vi "backwash.vi"(4 "Manual override":bool, 6 "Backwash control":T1, 8 "min filtration time [s]":dbl=600.0, 9 "Ripen time [s]":dbl=600.0, 10 "Filtered quality target [NTU]":dbl=0.3, 11 "Filtered Turbidity":dbl) -> (0 "backwashing?":i16, 1 "backwashing?":bool, 3 "last backwash":timestamp)   [LabVIEW 2019]
uses:
  Manual or Auto.ctl
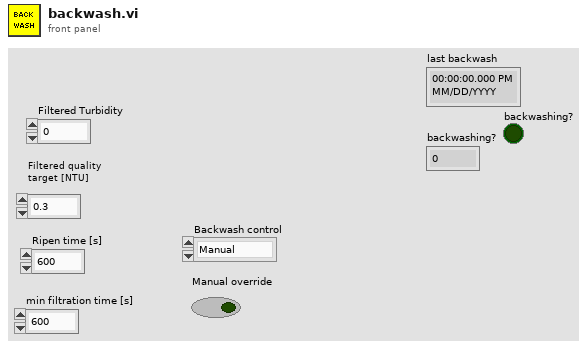
[diagram p1: front panel]
types:
  T1 = typedef "Manual or Auto.ctl" = enum16{"Manual", "Automatic"}
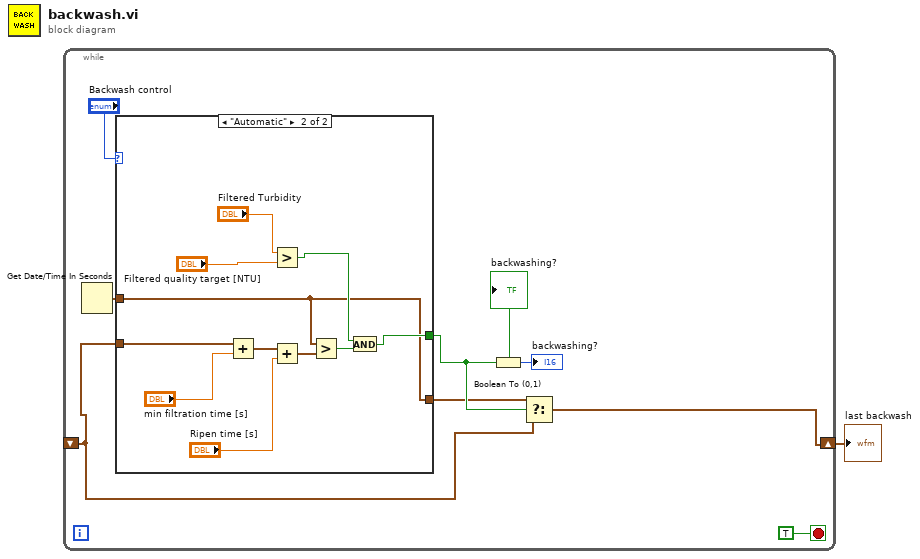
[diagram p0: block diagram]
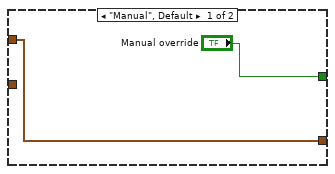
[diagram p2: hidden frame]
diagram:
  n1 = while {
    shift-right: [w8] -> w1
    shift-left: _ -> [w6]
    stop <- TRUE stop-if-true
    n2 = Get Date/Time In Seconds() -> (seconds since 1Jan1904=w5:timestamp)
    n3 = case shown="\"Automatic\"" "Backwash control" {
      tunnel: w6 -> [_ w15]
      tunnel: ["Manual override" w14] -> w3
      tunnel: w5 -> [w10 w12]
      tunnel: [w10 w12] -> w2
      frame "Manual", Default {
      }
      frame "Automatic" {
        n4 = Add(x=w15, y="min filtration time [s]") -> (x+y=w21:timestamp)
        n5 = Greater?(x="Filtered Turbidity", y="Filtered quality target [NTU]") -> (0:w13:bool)
        n6 = Add(x=w21, y="Ripen time [s]") -> (x+y=w18:timestamp)
        n7 = Greater?(x=w12, y=w18) -> (0:w20:bool)
        n8 = And(x=w13, y=w20) -> (x .and. y?=w14:bool)
      }
    }
    "backwashing?" <- w3
    n9 = Boolean To (0,1)(Boolean=w3) -> (0, 1=→"backwashing?":i16)
    n10 = Select(t=w2, s=w3, f=w6) -> (s? t:f=w8:timestamp)
  }
  "last backwash" <- w1
